vi "Z-scan_v2.vi"() -> ()   [LabVIEW 2010]
uses:
  <vilib>/Utility/error.llb/DialogType.ctl
  <vilib>/express/express arith-compare/Formula/XNode/ExpressFormulaBlockNode.xnode
  <vilib>/DAQmx/read.llb/DAQmx Read (Analog 1D Wfm NChan NSamp).vi
  <vilib>/DAQmx/create/channels.llb/DAQmx Create Channel (AI-Voltage-Basic).vi
  <vilib>/DAQmx/configure/timing.llb/DAQmx Timing (Sample Clock).vi
  <vilib>/DAQmx/configure/trigger.llb/DAQmx Start Trigger (Digital Edge).vi
  <vilib>/daqmx/miscellaneous.llb/DAQmx Fill In Error Info.vi
  <vilib>/express/express shared/transition.llb/Dynamic To Waveform Array.vi
  <vilib>/express/express shared/transition.llb/Waveform Array To Dynamic.vi
  <vilib>/express/express arith-compare/Formula/Block/exnFormulaBlock how many pts in the wave.vi
  <vilib>/express/express shared/ex_Modify Signal Name.vi
  C:/Arquivos de programas/National Instruments/LabVIEW 2010/resource/objmgr/daqmx.rc
panel:
  in  "error in":errorcluster
  in  "Tab Control 3":enum32{"Photodiode Signals", "Z-scan"}(tab)
  out "Trigger delay":dbl format="%#_6e"
  in  "stop 2":bool
  in  "Ring":u16(ring)=1 items=["Ref", "CA", "OA"]
  out "Signal 2":waveform(dbl)[](graph)
  in  "lower threshold":dbl
  in  "upper threshold":dbl
  out "Ioa":cluster{dbl[], dbl[]}(graph)
  out "Ica":cluster{dbl[], dbl[]}(graph)
  out "Ioca":cluster{dbl[], dbl[]}(graph)
  in  "z max (mm)":dbl=500.0
  in  "z step (mm)":dbl=5.0
  in  "N":i32=1000
  in  "z min (mm)":dbl=-0.5
  in  "stop 11":bool
  # "Config"
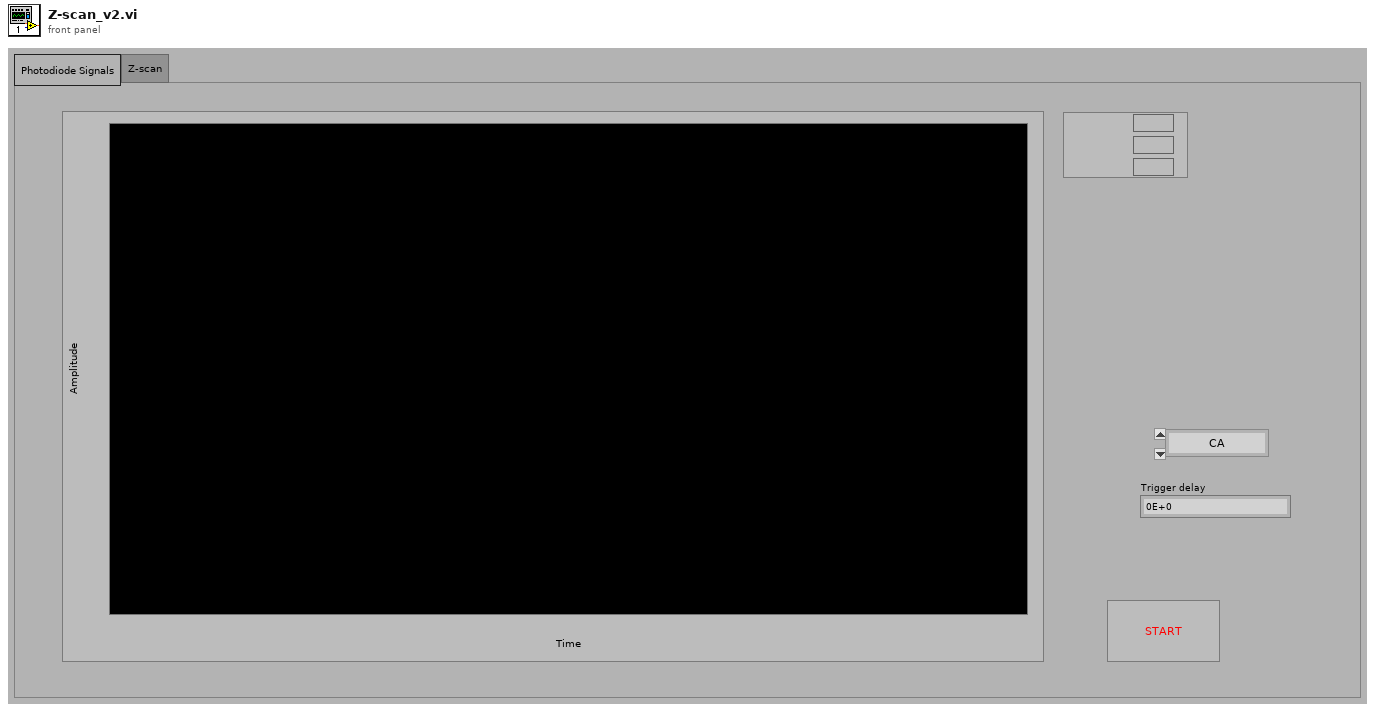
[diagram p1: front panel]
types:
  T1 = typedef "DialogType.ctl" = u16
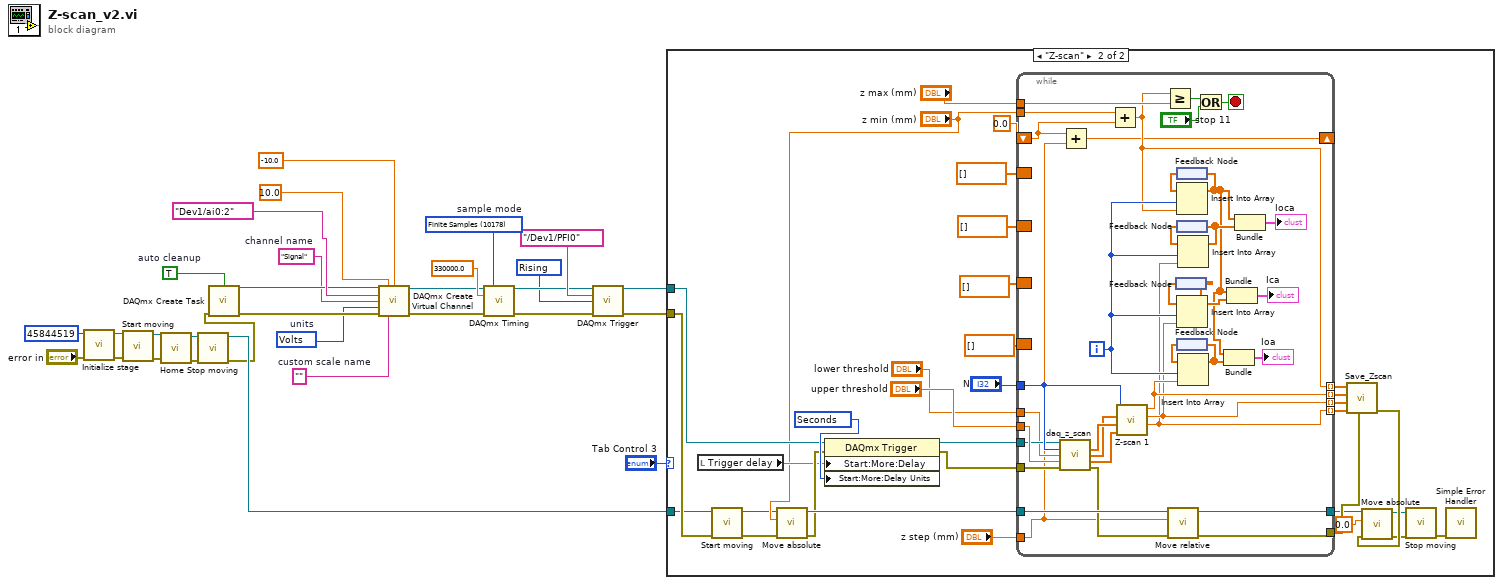
[diagram p0: block diagram]
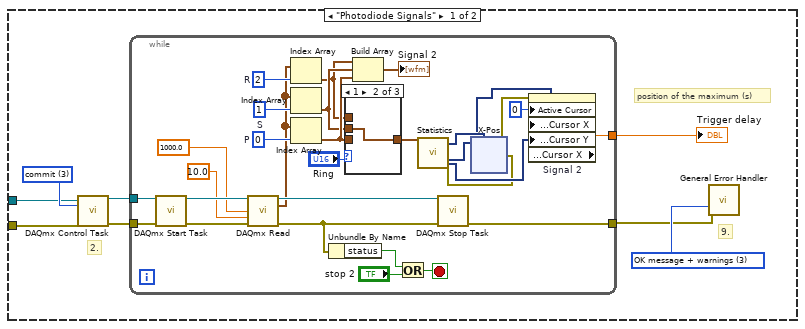
[diagram p2: hidden frame]
diagram:
  w20 = 10280 items=["Rising"=10280, "Falling"=10171] ("Trigger edge")
  w22 = 10178 items=["Finite Samples"=10178, "Continuous Samples"=10123, "Hardware Timed Single Point"=12522]  # sample mode
  w14 = 10348 items=["Volts"=10348, "From Custom Scale"=10065]  # units
  w15 = "Signal"  # channel name
  w13 = ""  # custom scale name
  w16 = TRUE  # auto cleanup
  n1 = call <userlib>:"Initialize stage.vi"("error in (no error)"="error in", "HWSerialNum"=45844519) -> ("error out"=w6:errorcluster, "reference out"=w8:refnum<k7>)  [unwired: 8 in]
  n2 = call <userlib>:"Start moving.vi"("error in (no error)"=w6, "Motor in"=w8) -> ("error out"=w5:errorcluster, "Motor out"=w7:refnum<k7>)  [unwired: 8 in]
  n3 = call <userlib>:"Home.vi"("error in"=w5, "in"=w7) -> ("error out"=w2:errorcluster, "out"=w4:refnum<k7>)  [unwired: 8 in]
  n4 = call <userlib>:"Stop moving.vi"("error in (no error)"=w2, "Motor in"=w4) -> ("error out"=w1:errorcluster, "Motor out"=w3:refnum<k7>)  [unwired: 8 in]
  n5 = call <vilib>:"DAQmx Create Task.vi"("auto cleanup"=w16, "error in"=w1) -> ("task out"=w17:refnum<k21>, "error out"=w19:errorcluster)  [unwired: 12 in]
  n6 = call-poly <vilib>:"DAQmx Create Virtual Channel.vi"("task in"=w17, "maximum value"=10.0 ("Maximum value (V)"), "minimum value"=-10.0 ("Minimum value (V)"), "physical channels"=tag "Dev1/ai0:2" ("Signal"), "name to assign"=w15, "units"=w14, "error in"=w19, "custom scale name"=w13) -> ("task out"=w27:refnum<k21>, "error out"=w28:errorcluster)  [unwired: 6 in]
  n7 = call-poly <vilib>:"DAQmx Timing.vi"("task/channels in"=w27, "sample mode"=w22, "rate"=330000.0, "error in"=w28) -> ("task out"=w21:refnum<k21>, "error out"=w24:errorcluster)  [unwired: 10 in]
  n8 = call-poly <vilib>:"DAQmx Trigger.vi"("task/channels in"=w21, "source"=tag "/Dev1/PFI0", "edge"=w20, "error in"=w24) -> ("task out"=w10:refnum<k21>, "error out"=w9:errorcluster)  [unwired: 10 in]
  n9 = case shown="\"Z-scan\"" "Tab Control 3" {
    tunnel: w10 -> [w32 w221]
    tunnel: w9 -> [w31 w214]
    tunnel: w3 -> [_ w213]
    frame "Photodiode Signals" {
      w38 = T1 3 items=["no dialog", "OK message", "continue or stop message", "OK message + warnings", "continue/stop + warnings"] ("type of dialog (OK msg:1)")
      w33 = 3 items=["verify"=2, "reserve"=4, "commit"=3, "unreserve"=5, "abort"=6] ("action")
      # "position of the maximum (s)"
      # "9."
      # "2."
      n10 = call <vilib>:"DAQmx Control Task.vi"("task/channels in"=w32, "action"=w33, "error in"=w31) -> ("task out"=w34:refnum<k21>, "error out"=w35:errorcluster)  [unwired: 11 in]
      n11 = while {
        tunnel: w34 -> [w68]
        tunnel: w35 -> [w67]
        tunnel: [w66] -> w37
        tunnel: [w44] -> w36
        stop <- w40 stop-if-true
        w59 = 0  # P
        w60 = 1  # S
        w61 = 2  # R
        n12 = call <vilib>:"DAQmx Start Task.vi"("task/channels in"=w68, "error in"=w67) -> ("task out"=w65:refnum<k21>, "error out"=w64:errorcluster)  [unwired: 12 in]
        n13 = call-poly <vilib>:"DAQmx Read.vi"("task/channels in"=w65, "number of samples per channel"=1000.0 ("Samples/channel"), "timeout"=10.0, "error in"=w64) -> ("task out"=w63:refnum<k21>, "data"=w58:waveform(dbl)[], "error out"=w42:errorcluster)  [unwired: 9 in]
        n14 = Index Array(array=w58, index=w61) -> (element=w50:waveform(dbl))
        n15 = Index Array(array=w58, index=w60) -> (element=w51:waveform(dbl))
        n16 = Index Array(array=w58, index=w59) -> (element=w53:waveform(dbl))
        n17 = Unbundle By Name(w42) -> ("status"=w43:bool)
        n18 = case shown="1" "Ring" {
          tunnel: w53 -> [w208 _ _]
          tunnel: [w208 w209 w210] -> w52
          tunnel: w51 -> [_ w209 _]
          tunnel: w50 -> [_ _ w210]
          frame 0, Default {
          }
          frame 1 {
          }
          frame 2 {
          }
        }
        n19 = Build Array(w50, w51, w53) -> (→"Signal 2":waveform(dbl)[])
        n20 = Or(x=w43, y="stop 2") -> (x .or. y?=w40:bool)
        n21 = call "Statistics"("Signals"=w52) -> ("First Time"=w55:dynamicdata, "Time of Maximum"=w56:dynamicdata, "Maximum"=w54:dynamicdata, "error out"=w49:errorcluster)  [unwired: 21 in, 2 out]
        n22 = call <vilib>:"DAQmx Stop Task.vi"("task/channels in"=w63, "error in"=w42) -> ("error out"=w44:errorcluster)  [unwired: 12 in, 1 out]
        n23 = xnode "X-Pos"("TimeMax"=w56, "1stTime"=w55, "error in (no error)"=w49) -> ("Result"=w45:dynamicdata, "error out"=w48:errorcluster)
        n24 = property on="Signal 2" class="WFGraph (strict)"(error in=w48, "Active Cursor"=u32 0, "Cursor.Cursor Position:Cursor X"=w45, "Cursor.Cursor Position:Cursor Y"=w54) -> ("Cursor.Cursor Position:Cursor X"=w66:dbl)  [unwired: 1 in, 2 out]
      }
      "Trigger delay" <- w37
      n25 = call <vilib>:"General Error Handler.vi"("type of dialog (OK msg:1)"=w38, "error in (no error)"=w36) -> ()  [unwired: 9 in, 5 out]
    }
    frame "Z-scan" {
      w233 = 10364 items=["Sample Clock Periods"=10286, "Seconds"=10364, "Ticks"=10304] ("Start.DelayUnits")
      n26 = local read "Trigger delay"() -> (w223:dbl)
      n27 = call <userlib>:"Start moving.vi"("error in (no error)"=w214, "Motor in"=w213) -> ("error out"=w211:errorcluster, "Motor out"=w212:refnum<k7>)  [unwired: 8 in]
      n28 = call <userlib>:"Move absolute.vi"("error in (no error)"=w211, "target position"="z min (mm)", "Motor in"=w212) -> ("error out"=w229:errorcluster, "Motor out"=w230:refnum<k7>)  [unwired: 7 in]
      n29 = property class="DAQmx Trigger"(reference=w221, error in=w229, "Start:More:Delay"=w223, "Start:More:Delay Units"=w233) -> (reference out=w232:refnum<k21>, error out=w231:errorcluster)
      n30 = while {
        tunnel: "z max (mm)" -> [w277]
        tunnel: [w253] -> w224
        tunnel: "z min (mm)" -> [w273]
        tunnel: "z step (mm)" -> [w251]
        tunnel: w230 -> [w271]
        tunnel: "N" -> [w272]
        shift-right: [w252] -> _
        shift-left: 0.0 -> [w268]
        border: dbl[] [] -> [_]
        tunnel: w231 -> [w255]
        tunnel: "upper threshold" -> [w270]
        tunnel: w232 -> [w269]
        border: dbl[] [] -> [_]
        border: dbl[] [] -> [_]
        border: dbl[] [] -> [_]
        tunnel: [w257] -> w228 mode=indexing
        tunnel: "lower threshold" -> [w256]
        tunnel: [w247] -> w227 mode=indexing
        tunnel: [w246] -> w226 mode=indexing
        tunnel: [w245] -> w225 mode=indexing
        tunnel: [w244] -> w220
        i -> [w261]
        stop <- w275 stop-if-true
        n31 = call <userlib>:"daq_z_scan.vi"("channels in"=w269, "N"=w272, "lower threshold"=w256, "upper threshold"=w270, "error in"=w255) -> ("CA"=w267:dbl[], "OA"=w266:dbl[], "Ref"=w265:dbl[], "error out"=w254:errorcluster)  [unwired: 6 in, 1 out]
        n32 = Add(x=w268, y=w251) -> (x+y=w252:dbl)
        n33 = Add(x=w273, y=w268) -> (x+y=w257:dbl)
        n34 = call <userlib>:"Z-scan 1.vi"("Ref"=w265, "CA"=w267, "OA"=w266, "N"=w272) -> ("Ioca"=w245:dbl, "Ica"=w246:dbl, "Ioa"=w247:dbl)  [unwired: 3 in]
        n35 = Greater Or Equal?(x=w257, y=w277) -> (x >= y?=w276:bool)
        n36 = call <userlib>:"Move relative.vi"("error in (no error)"=w254, "target position"=w251, "Motor in"=w271) -> ("error out"=w253:errorcluster, "Motor out"=w244:refnum<k7>)  [unwired: 7 in]
        n37 = feedback #1() -> (w264:dbl[])
        n38 = feedback #2() -> (w260:dbl[])
        n39 = Insert Into Array(array=w260, index=w261, new element=w257) -> (w250:dbl[])
        n40 = feedback-in #2(w250) -> ()
        n41 = feedback #3() -> (w259:dbl[])
        n42 = Insert Into Array(array=w264, index=w261, new element=w246) -> (w263:dbl[])
        n43 = feedback-in #1(w263) -> ()
        n44 = feedback #4() -> (w279:dbl[])
        n45 = Insert Into Array(array=w259, index=w261, new element=w245) -> (w262:dbl[])
        n46 = feedback-in #3(w262) -> ()
        n47 = Insert Into Array(array=w279, index=w261, new element=w247) -> (w278:dbl[])
        n48 = feedback-in #4(w278) -> ()
        n49 = Or(x=w276, y="stop 11") -> (x .or. y?=w275:bool)
        n50 = Bundle(w250, w278) -> (→"Ioa":cluster{dbl[], dbl[]})  [unwired: 1 in]
        n51 = Bundle(w250, w263) -> (→"Ica":cluster{dbl[], dbl[]})  [unwired: 1 in]
        n52 = Bundle(w250, w262) -> (→"Ioca":cluster{dbl[], dbl[]})  [unwired: 1 in]
      }
      n53 = call "Save_Zscan.vi"("error in"=w224, "Ioca"=w225, "Ica"=w226, "Ioa"=w227, "z (mm)"=w228) -> ("error out"=w219:errorcluster)  [unwired: 6 in]
      n54 = call <userlib>:"Move absolute.vi"("error in (no error)"=w219, "target position"=sgl 0.0 ("Set absolute position"), "Motor in"=w220) -> ("error out"=w218:errorcluster, "Motor out"=w217:refnum<k7>)  [unwired: 7 in]
      n55 = call <userlib>:"Stop moving.vi"("error in (no error)"=w218, "Motor in"=w217) -> ("error out"=w222:errorcluster)  [unwired: 8 in, 1 out]
      n56 = call <vilib>:"Simple Error Handler.vi"("error in (no error)"=w222) -> ()  [unwired: 1 in, 8 out]
    }
  }
